vi "Read Batch Profiles.vi"(8 "error in (no error)":errorcluster {"code" format="%.0x"}, 9 "Data Size (0: Auto Size)":u32, 10 "Read Batch Profile Req":T2 {"Batch Pos" items=["CURRENT"=0, "SPECIFY"=2, "COMMITED"=3, "NEWEST PROFILE"=4]}, 11 "Device ID (0)":i32) -> (0 "error out":errorcluster {"code" format="%.0x"}, 1 "Read Batch Profile Rsp":T1, 2 "Profile Data":u32[](array[numeric]), 3 "Device ID out":i32, 5 "Profile Info":T4)   [LabVIEW 2020, in "KEYENCE LJ-X8000A.lvlib"]
doc: "This function gets profile data when bacth measurement is ON.\nProfile data is stored in units of 0.01 ƒÊm.\nFor details on the data stored in the profile data, refer to the reference manual."
uses:
  KEYENCE LJ-X8000A.lvlib
  Clusters/Profile Info.ctl
  Clusters/Read Batch Profile Req.ctl
  Constants/Batch Pos.ctl
  Clusters/Read Batch Profile Rsp.ctl
panel:
  # "(c) 2019 KEYENCE CORPORATION.  ALL RIGHTS RESERVED."
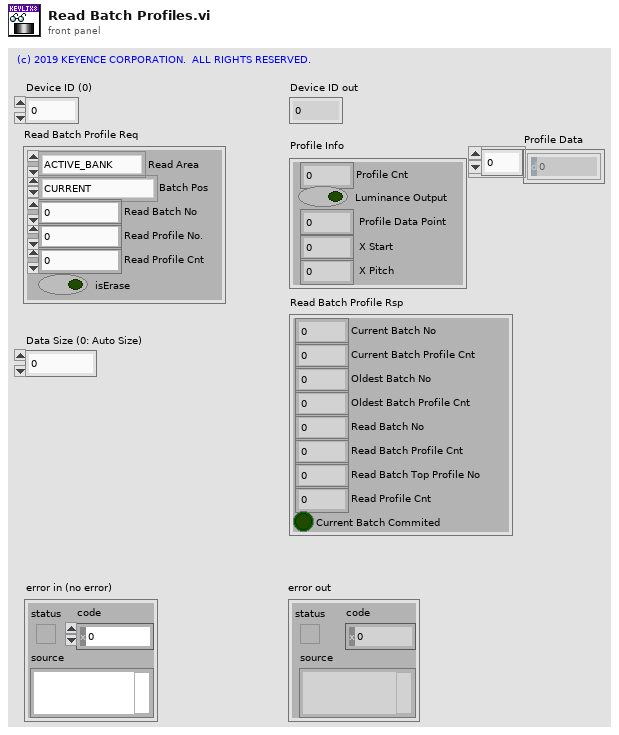
[diagram p1: front panel]
types:
  T1 = typedef "KEYENCE LJ-X8000A.lvlib/Read Batch Profile Rsp.ctl" = cluster{"Current Batch No":u32, "Current Batch Profile Cnt":u32, "Oldest Batch No":u32, "Oldest Batch Profile Cnt":u32, "Read Batch No":u32, "Read Batch Profile Cnt":u32, "Read Batch Top Profile No":u32, "Read Profile Cnt":u32, "Current Batch Commited":bool}
  T2 = typedef "KEYENCE LJ-X8000A.lvlib/Read Batch Profile Req.ctl" = cluster{"Read Area":enum8{"ACTIVE_BANK", "INACTIVE_BANK"}, "Batch Pos":T3, "Read Batch No":u32, "Read Profile No.":u32, "Read Profile Cnt":u8, "isErase":bool}
  T3 = typedef "KEYENCE LJ-X8000A.lvlib/Batch Pos.ctl" = u8
  T4 = typedef "KEYENCE LJ-X8000A.lvlib/Profile Info.ctl" = cluster{"Profile Cnt":u8, "Luminance Output":bool, " Profile Data Point":u16, " X Start":i32, " X Pitch":i32}
  T5 = cluster{"byTargetBank":u8, "Batch Pos":T3, "reserve":u8, "reserve":u8, "dwGetBatchNo":u32, "dwGetProfileNo":u32, "byGetProfileCount":u8, "byErase":u8, "reserve":u8, "reserve":u8}
  T6 = cluster{"byProfileCount":u8, "reserve":u8, "byLuminanceOutput":u8, "reserve":u8, "wProfileDataCount":u16, "reserve":u8, "reserve":u8, "lXStart":i32, "lXPitch":i32}
  T7 = cluster{"dwCurrentBatchNo":u32, "dwCurrentBatchProfileCount":u32, "dwOldestBatchNo":u32, "dwOldestBatchProfileCount":u32, "dwGetBatchNo":u32, "dwGetBatchProfileCount":u32, "dwGetBatchTopProfileNo":u32, "byGetProfileCount":u8, "byCurrentBatchCommited":u8, "reserve":u8, "reserve":u8}
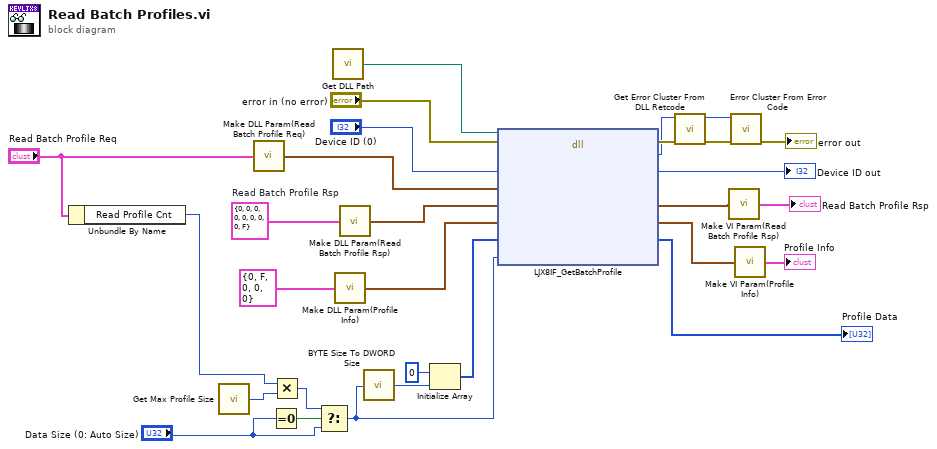
[diagram p0: block diagram]
diagram:
  w6 = T1 {"Current Batch No"=0, "Current Batch Profile Cnt"=0, "Oldest Batch No"=0, "Oldest Batch Profile Cnt"=0, "Read Batch No"=0, "Read Batch Profile Cnt"=0, "Read Batch Top Profile No"=0, "Read Profile Cnt"=0, "Current Batch Commited"=FALSE}  # Read Batch Profile Rsp
  n1 = Unbundle By Name("Read Batch Profile Req") -> ("Read Profile Cnt"=w9:u8)
  n2 = call "Get Max Profile Size.vi"() -> ("Profile Size"=w22:u32)  [unwired: 5 in]
  n3 = call "Make DLL Param(Read Batch Profile Req).vi"("Read Batch Profile Req"="Read Batch Profile Req") -> ("pReq"=w7:T5)
  n4 = Equal To 0?(x="Data Size (0: Auto Size)") -> (x = 0?=w23:bool)
  n5 = Multiply(x=w9, y=w22) -> (x*y=w21:u32)
  n6 = Select(t=w21, s=w23, f="Data Size (0: Auto Size)") -> (s? t:f=w10:u32)
  n7 = call "Get DLL Path.vi"() -> ("DLL Path"=w27:path)  [unwired: 3 in]
  n8 = call "Make DLL Param(Profile Info).vi"("Profile Info"=T4 {"Profile Cnt"=0, "Luminance Output"=FALSE, " Profile Data Point"=0, " X Start"=0, " X Pitch"=0}) -> ("DLL Parameter"=w15:T6)
  n9 = call "Make DLL Param(Read Batch Profile Rsp).vi"("Read Batch Profile Rsp"=w6) -> ("pRsp"=w5:T7)
  n10 = call "BYTE Size To DWORD Size.vi"("BYTE Size"=w10) -> ("DWORD Size"=w11:u32)
  n11 = Initialize Array(u32 0, w11) -> (w19:u32[])
  n12 = dll-call lib="C:/Program Files (x86)/National Instruments/LabVIEW 2018/instr.lib/KEYENCE LJ-X8000/LJX8_IF.*" fn="LJX8IF_GetBatchProfile"(path in=w27, error in="error in (no error)", "lDeviceId"="Device ID (0)", "pReq"=w7, "pRsp"=w5, "pProfileInfo"=w15, "pdwProfileData"=w19, "dwDataSize"=w10) -> (error out=w18:errorcluster, "lRetCode"=w17:i32, "lDeviceId"=→"Device ID out":i32, "pRsp"=w4:T7, "pProfileInfo"=w13:T6, "pdwProfileData"=→"Profile Data":u32[])  [unwired: 3 in, 1 out]
  n13 = call "Get Error Cluster From DLL Retcode.vi"("error in (no error)"=w18, "DLL Return Code"=w17) -> ("error out"=w16:errorcluster, "VI Error Code"=w1:i32)  [unwired: 8 in]
  n14 = call "Make VI Param(Read Batch Profile Rsp).vi"("pRsp"=w4) -> ("Read Batch Profile Rsp"=→"Read Batch Profile Rsp":T1)
  n15 = call <vilib>:"Error Cluster From Error Code.vi"("error in (no error)"=w16, "error code (0)"=w1) -> ("error out"=→"error out":errorcluster)  [unwired: 7 in]
  n16 = call "Make VI Param(Profile Info).vi"("pProfileInfo"=w13) -> ("Profile Info"=→"Profile Info":T4)
